vi "Untitled 4.vi"() -> ()   [LabVIEW 2018]
uses:
  <vilib>/measure/NI_MABase.lvlib
panel:
  out "Numeric":u32
  in  "stop":bool
  out "Waveform Chart":waveform(dbl)(graph)
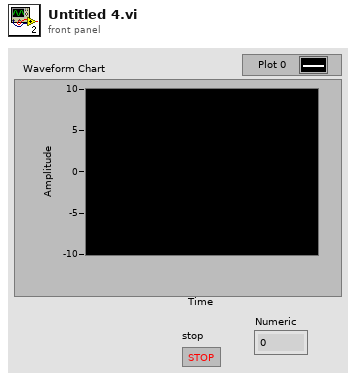
[diagram p1: front panel]
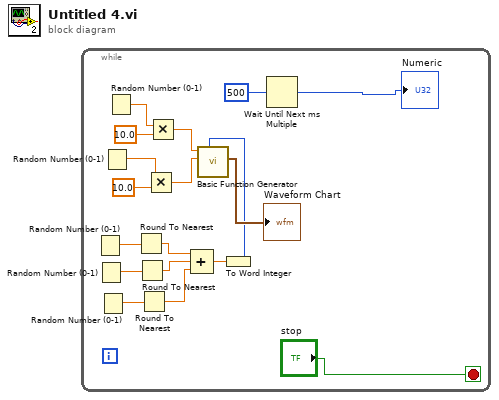
[diagram p0: block diagram]
diagram:
  n1 = while {
    stop <- "stop" stop-if-true
    n2 = Random Number (0-1)() -> (number: 0 to 1=w9:dbl)
    n3 = Random Number (0-1)() -> (number: 0 to 1=w8:dbl)
    n4 = Random Number (0-1)() -> (number: 0 to 1=w7:dbl)
    n5 = Random Number (0-1)() -> (number: 0 to 1=w15:dbl)
    n6 = Random Number (0-1)() -> (number: 0 to 1=w16:dbl)
    n7 = Round To Nearest(number=w9) -> (nearest integer value=w6:dbl)
    n8 = Round To Nearest(number=w8) -> (nearest integer value=w5:dbl)
    n9 = Round To Nearest(number=w7) -> (nearest integer value=w4:dbl)
    n10 = Multiply(x=w15, y=10.0) -> (x*y=w13:dbl)
    n11 = Multiply(x=w16, y=10.0) -> (x*y=w14:dbl)
    n12 = Compound Arithmetic op=ADD(w6, w5, w4) -> (w3:dbl)
    n13 = To Word Integer(number=w3) -> (16bit integer=w2:i16)
    n14 = call <vilib>:"Basic Function Generator.vi"("signal type"=w2, "amplitude"=w13, "frequency"=w14) -> ("signal out"=→"Waveform Chart":waveform(dbl))  [unwired: 6 in, 2 out]
    n15 = Wait Until Next ms Multiple(millisecond multiple=u32 500) -> (millisecond timer value=→"Numeric":u32)
  }
